vi "QI_GetCamInfo.vi"(7 "path to dll":path, 8 "error in (no error)":errorcluster, 10 "paramKey":u32, 11 "Camera Handle":u32) -> (0 "error out":errorcluster, 1 "CamInfo err":i32, 2 "paramVal":u32, 3 "Camera Handle":u32)   [LabVIEW 2014]
panel:
  in  "paramVal":u32
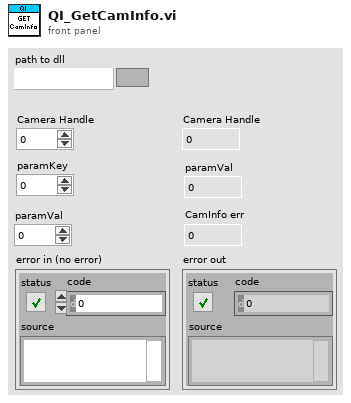
[diagram p1: front panel]
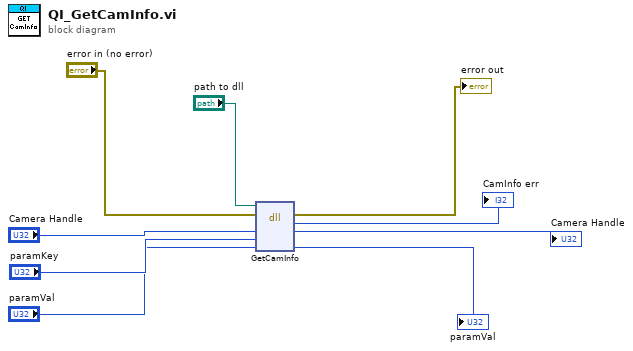
[diagram p0: block diagram]
diagram:
  n1 = dll-call lib="C:/Users/appli/Documents/Aline/octo-labview/QImaging/Release/QImaging.dll" fn="GetCamInfo"(path in="path to dll", error in="error in (no error)", "handle"="Camera Handle", "paramKey"="paramKey", "paramVal"="paramVal") -> (error out=→"error out":errorcluster, "return type"=→"CamInfo err":i32, "handle"=→"Camera Handle":u32, "paramVal"=→"paramVal":u32)  [unwired: 2 in, 1 out]
